vi "[MAIN] Image To IMAQ LV2012 NIVerified.vi"() -> ()   [LabVIEW 2018]
doc: "This VI demonstrates how you can use the <b>Convert LabVIEW Image Data To IMAQ.VI<b>."
uses:
  Instance           1 33Saved   Front Panel Image to IMAQ .vi
panel:
  out "Image":T1(plugin-control)
  out "Sine":dynamicdata(graph)
  # "Overview: Demonstrates how to convert LabVIEW Image data into IMAQ Image data. \nRequirements: LabVIEW Base Development System 2012 (or compatible)\n                             NI Vision Development Module 2012 (or compatible)\nInstructions: \n1. Run the VI."
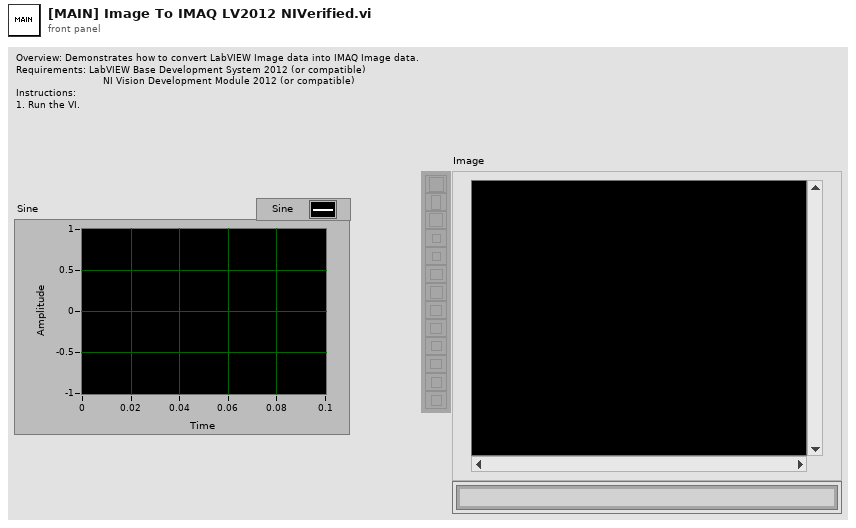
[diagram p1: front panel]
types:
  T1 = typedef "IMAQ Image.ctl" = refnum<image>
  T2 = typedef "Image Type" = u32
  T3 = typedef "imagedata.ctl" = cluster{"image type":i32, "image depth":i32, "image":u8[], "mask":u8[], "colors":u32[], "Rectangle":cluster{"left":i16, "top":i16, "right":i16, "bottom":i16}}
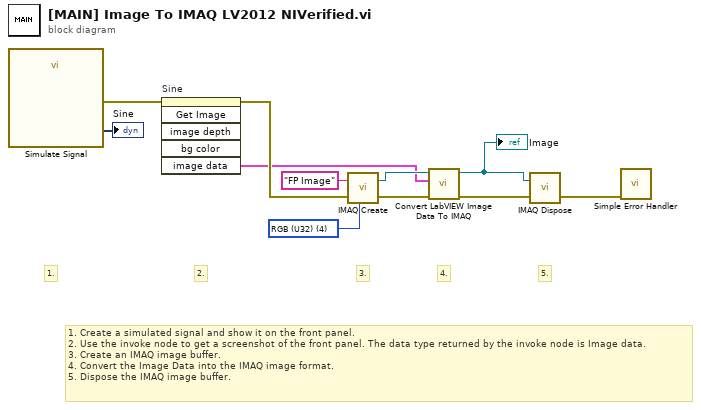
[diagram p0: block diagram]
diagram:
  w8 = T2 4 items=["Grayscale (U8)", "Grayscale (I16)", "Grayscale (SGL)", "Complex (CSG)", "RGB (U32)", "HSL (U32)", "RGB (U64)", "Grayscale (U16)"] ("Image Type")
  # "5."
  # "4."
  # "3."
  # "2."
  # "1."
  # "1. Create a simulated signal and show it on the front panel.\n2. Use the invoke node to get a screenshot of the front panel. The data type returned by the invoke node is Image data.\n3. Create an IMAQ image buffer.\n4. Convert the Image Data into the IMAQ image format.\n5. Dispose the IMAQ image buffer."
  n1 = call "Simulate Signal"() -> ("Sine"=→"Sine":dynamicdata, "error out"=w10:errorcluster)  [unwired: 14 in]
  n2 = invoke on="Sine" class="WFGraph (strict)" method="Get Image"(error in=w10) -> (error out=w7:errorcluster, "image data"=w4:T3)  [unwired: 5 in, 4 out]
  n3 = call "IMAQ Create"("Image Name"="FP Image", "Image Type"=w8, "error in (no error)"=w7) -> ("New Image"=w5:T1, "error out"=w6:errorcluster)  [unwired: 2 in]
  n4 = call "Convert LabVIEW Image Data To IMAQ.vi"("error in (no error)"=w6, "Image Data"=w4, "Image In"=w5) -> ("error out"=w3:errorcluster, "Image Out"=w2:T1)  [unwired: 7 in]
  "Image" <- w2
  n5 = call "IMAQ Dispose"("Image"=w2, "error in (no error)"=w3) -> ("error out"=w1:errorcluster)  [unwired: 4 in]
  n6 = call <vilib>:"Simple Error Handler.vi"("error in (no error)"=w1) -> ()  [unwired: 4 in, 5 out]
